vi "Convert TCP Mode.vi"(10 "Mode":T2) -> (2 "TCP Mode":T1(ring))   [LabVIEW 2020, in "Stream-TCP.lvlib" / "TCP Stream.lvclass"]
uses:
  TCP Stream.lvclass
  <vilib>/IlluminatedG/lv-stream/stream/Mode.ctl
  <vilib>/IlluminatedG/lv-stream/Stream.lvlib
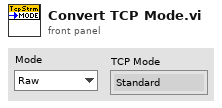
[diagram p1: front panel]
types:
  T1 = enum16{"Standard", "Buffered", "CRLF", "Immediate"}
  T2 = typedef "Stream.lvlib/Mode.ctl" = enum16{"Raw", "Buffered", "LineTerm"}
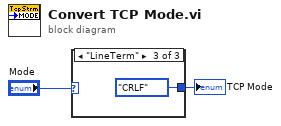
[diagram p0: block diagram]
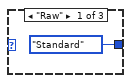
[diagram p2: hidden frame]
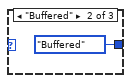
[diagram p3: hidden frame]
diagram:
  n1 = case shown="\"LineTerm\"" "Mode" {
    tunnel: [T1."Standard" ("mode") T1."Buffered" ("mode") T1."CRLF" ("mode")] -> w1
    frame "Raw" {
    }
    frame "Buffered" {
    }
    frame "LineTerm" {
    }
  }
  "TCP Mode" <- w1
